vi "Get Intensity Graph Value.vi"(8 "error in (no error)":errorcluster, 11 "graph_utilities in":refnum<class "graph_utilities.lvclass">) -> (0 "error out":errorcluster, 2 "Value":dbl[][](array[numeric]), 3 "graph_utilities out":refnum<class "graph_utilities.lvclass">)   [LabVIEW 2020, in "graph_utilities.lvclass"]
doc: "Get the current value of the Intensity Graph"
uses:
  graph_utilities.lvclass
  graph_utilities.lvclass/graph_utilities.ctl
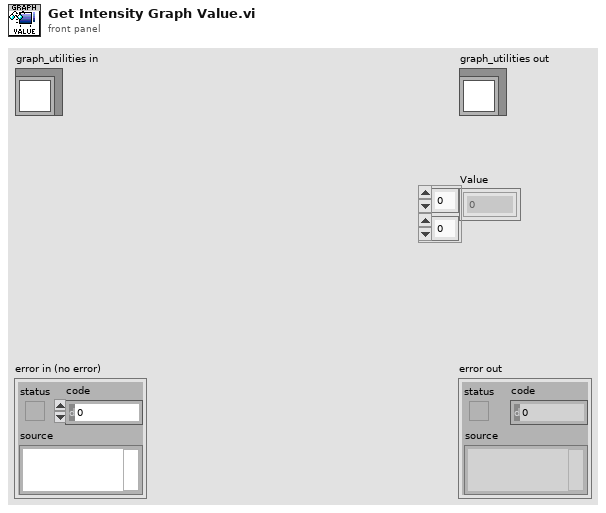
[diagram p1: front panel]
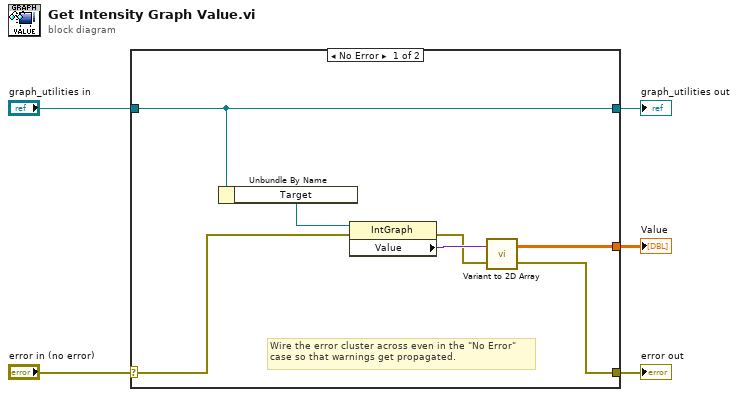
[diagram p0: block diagram]
diagram:
  n1 = case shown="No Error" "error in (no error)" {
    selector: "error in (no error)" -> [w6 w14]
    tunnel: [w9 w14] -> w4
    tunnel: [w12 w13] -> w2
    tunnel: "graph_utilities in" -> [w12 w13]
    tunnel: [w10 _] -> w1
    frame No Error {
      # "Wire the error cluster across even in the \"No Error\"\ncase so that warnings get propagated."
      n2 = Unbundle By Name(w12) -> ("Target"=w7:refnum<vi>)
      n3 = property on="Property Node" class="IntGraph"(reference=w7, error in=w6) -> (error out=w8:errorcluster, "Value"=w11:variant)  [unwired: 1 out]
      n4 = call "Variant to 2D Array.vi"("error in (no error)"=w8, "Value"=w11) -> ("error out"=w9:errorcluster, "Array"=w10:dbl[][])
    }
    frame Error {
    }
  }
  "error out" <- w4
  "graph_utilities out" <- w2
  "Value" <- w1
